vi "Autonomous Independent.vi"() -> ()   [LabVIEW 2014]
doc: "This VI is called when autonomous begins, and will automatically be terminated when autonomous ends. You can carry out timed or sensor driven robot movement independently without needing to return to the caller."
uses:
  <vilib>/Rock Robotics/WPI/Joystick/WPI_JoystickGetSetRefNum.vi
  <vilib>/Rock Robotics/Network Tables/SD Write Numeric Array.vi
  <vilib>/Rock Robotics/WPI/RobotDrive/WPI_RobotDriveGetSetRefNum.vi
  <vilib>/Rock Robotics/WPI/RobotDrive/WPI_RobotDriveMecanumDrive_Cartesian.vi
panel:
  out "Current Movement, for debugging":T1 {"Z Joystick Value" scale=-1.0..1.0; "Y Joystick Value" scale=1.0..-1.0; "X Joystick Value" scale=-1.0..1.0}
  in  "Array of robot movements":T2(array[cluster]) {"Z Joystick Value" scale=-1.0..1.0; "Y Joystick Value" scale=1.0..-1.0; "X Joystick Value" scale=-1.0..1.0}
  # "Be sure to right-click and choose Data Operations>>Make Current Value default if you want to save the array values with the VI"
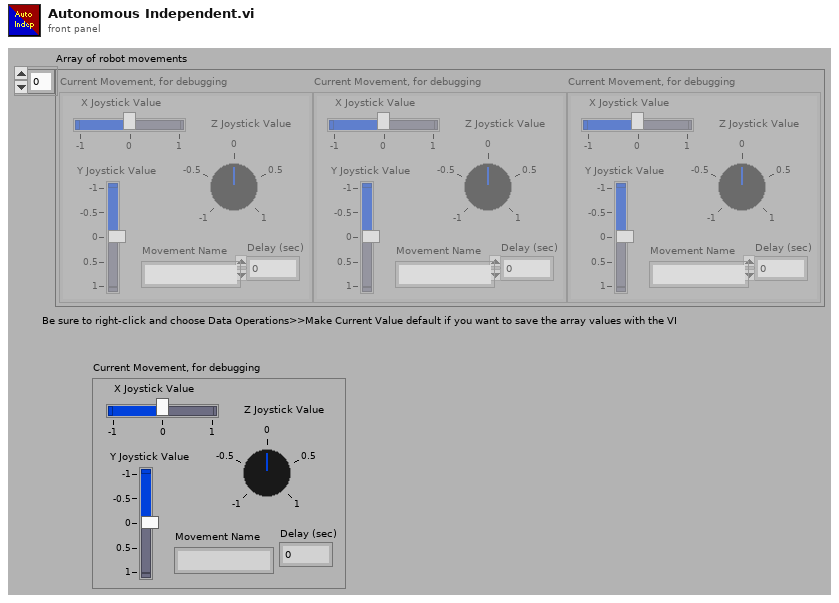
[diagram p1: front panel]
types:
  T1 = cluster{"X Joystick Value":dbl, "Y Joystick Value":dbl, "Z Joystick Value":dbl, "Delay (sec)":dbl, "Movement Name":string}
  T2 = cluster{"X Joystick Value":dbl, "Y Joystick Value":dbl, "Z Joystick Value":dbl, "Delay (sec)":dbl, "Movement Name":string}[]
  T3 = typedef "WPI_MotorControlDeviceRef.ctl" = cluster{"DeviceStatus":errorcluster, "Type":T4, "PWM":cluster{"Controller":T5, "PWM Channel":T6, "DeadBand":T7}, "CAN":cluster{"Device Number":u8, "Control Mode":T8, "Semaphore":T9, "Max Vout":dbl, "TalonSRX Control Mode":T10}, "Invert":bool, "TransformRef":T11, "InvTransformRef":T11}
  T4 = typedef "WPI_MotorControlType.ctl" = enum16{"PWM", "CAN", "CANTalonSRX"}
  T5 = typedef "FPGA_TypedefDigitalModule.ctl" = enum16{"Controller 1"}
  T6 = typedef "FPGA_DIOPWMChannel.ctl" = enum8{"PWM 0", "PWM 1", "PWM 2", "PWM 3", "PWM 4", "PWM 5", "PWM 6", "PWM 7", "PWM 8", "PWM 9", "PWM MXP 0", "PWM MXP 1", "PWM MXP 2", "PWM MXP 3", "PWM MXP 4", "PWM MXP 5", "PWM MXP 6", "PWM MXP 7", "PWM MXP 8", "PWM MXP 9", "Invalid"}
  T7 = typedef "WPI_PWMDeadband.ctl" = cluster{"Name":string, "maxPositivePwm":i32, "minPositivePwm":i32, "centerPwm":i32, "maxNegativePwm":i32, "minNegativePwm":i32, "angularRange":u16}
  T8 = typedef "WPI_CANJaguar_ControlMode.ctl" = enum8{"Percent VBus", "Current", "Speed", "Position", "Voltage"}
  T9 = typedef "Semaphore RefNum" = refnum<k1>
  T10 = typedef "WPI_CANTalonSRX_APIControlMode.ctl" = enum8{"Percent VBus", "Speed", "Position", "Slave", "Unchanged / Invalid"}
  T11 = typedef "WPI_PWMTransform_ConPane.ctl" = refnum<vi>
  T12 = typedef "WPI_RobotDriveDevRef.ctl" = cluster{"DevStatus":errorcluster, "Motors[]":T3[], "Square Inputs":bool, "Max Output":dbl}
  T13 = typedef "WPI_JoystickDevRef.ctl" = cluster{"Device":T14}
  T14 = typedef "WPI_JoystickDeviceEnum.ctl" = enum16{"USB 0", "USB 1", "USB 2", "USB 3", "USB 4", "USB 5"}
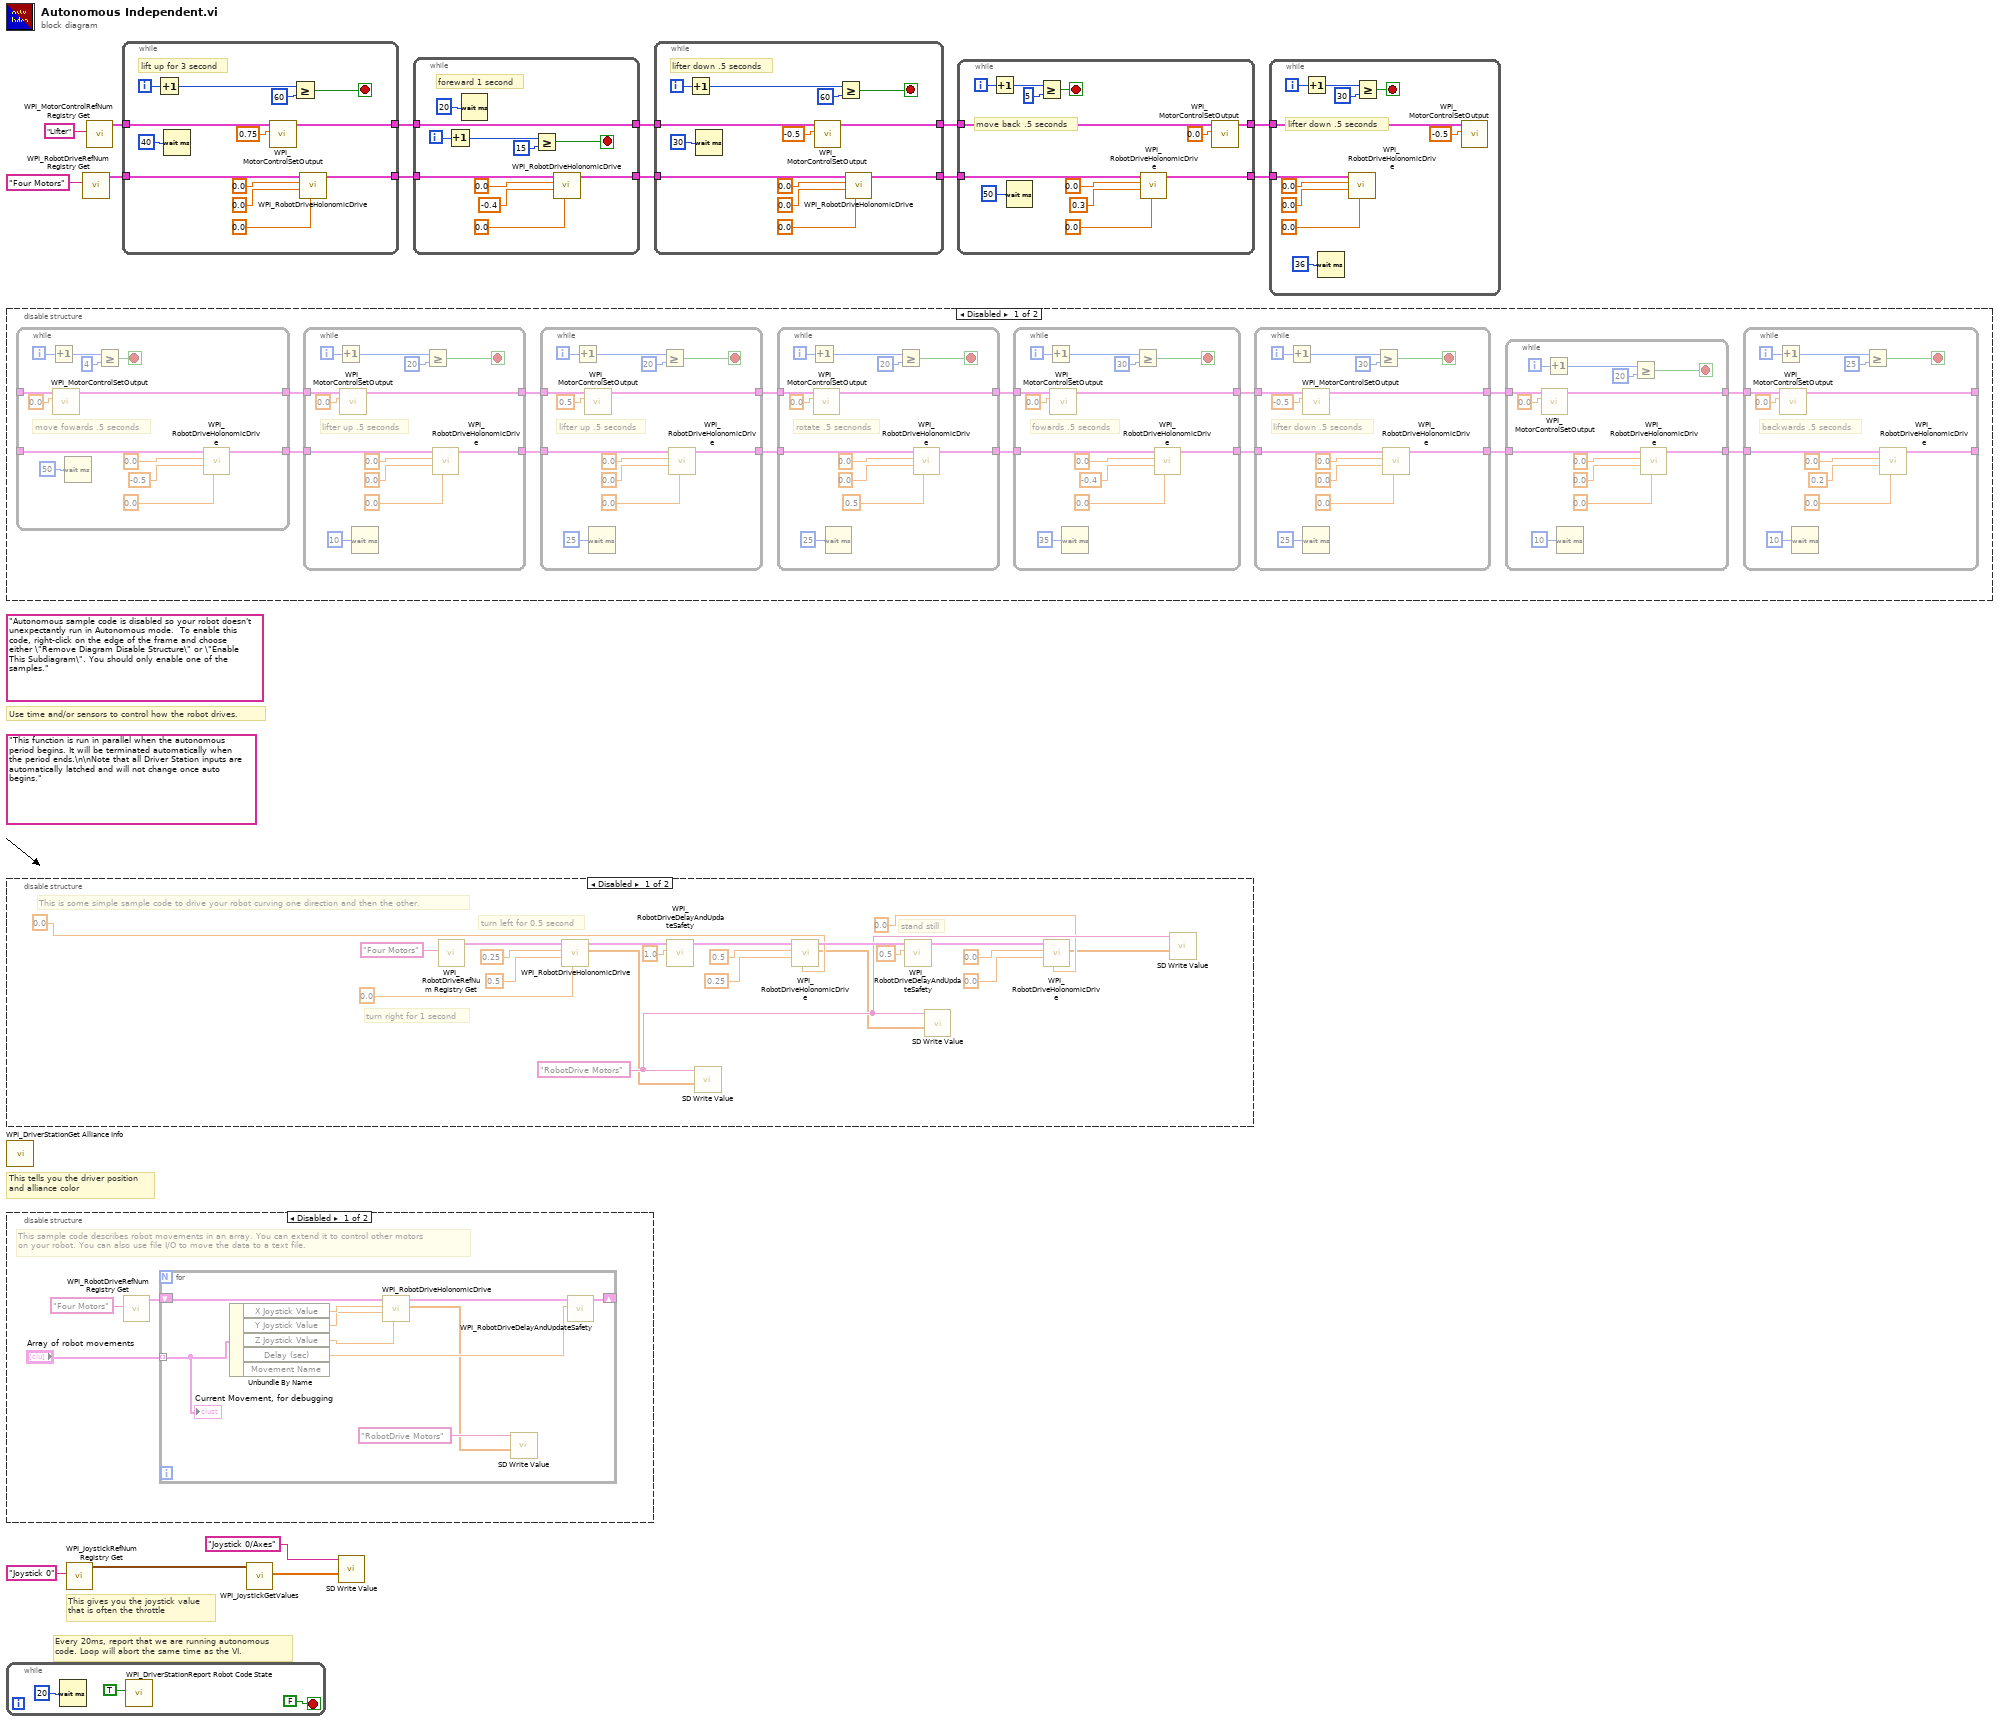
[diagram p0: block diagram]
diagram:
  (unwired) "Autonomous sample code is disabled so your robot doesn't unexpectantly run in Autonomous mode.  To enable this code, right-click on the edge of the frame and choose either \"Remove Diagram Disable Structure\" or \"Enable This Subdiagram\". You should only enable one of the samples."
  (unwired) "This function is run in parallel when the autonomous period begins. It will be terminated automatically when the period ends.\n\nNote that all Driver Station inputs are automatically latched and will not change once auto begins."
  # "Every 20ms, report that we are running autonomous\ncode. Loop will abort the same time as the VI."
  # "This gives you the joystick value\nthat is often the throttle"
  # "Use time and/or sensors to control how the robot drives."
  # "This tells you the driver position\nand alliance color"
  n1 = disable-structure shown="Disabled" {
    frame Disabled {
      n2 = while {
        tunnel: [w117] -> w19
        tunnel: [w113] -> w20
        tunnel: _ -> [w110]
        tunnel: _ -> [w109]
        i -> [w119]
        stop <- w118 stop-if-true
        # "move fowards .5 seconds"
        n3 = Increment(x=w119) -> (x+1=w120:i32)
        n4 = call <vilib>:"WPI_MotorControlSetOutput.vi"("Output"=0.0, "MotorControlDevRef"=w109) -> ("MotorControlDevRef"=w113:T3)  [unwired: 7 in, 2 out]
        n5 = Wait (ms)(milliseconds to wait=u32 50) -> ()  [unwired: 1 out]
        n6 = Greater Or Equal?(x=w120, y=4) -> (x >= y?=w118:bool)
        n7 = call-poly <vilib>:"WPI_RobotDriveHolonomicDrive.vi"("Rotation"=0.0, "Y"=-0.5 ("X"), "X"=0.0 ("Y"), "RobotDriveDevRef"=w110) -> ("RobotDriveDevRef"=w117:T12)  [unwired: 5 in, 2 out]
      }
      n8 = while {
        tunnel: [w130] -> w21
        tunnel: [w126] -> w22
        tunnel: w20 -> [w123]
        tunnel: w19 -> [w122]
        i -> [w132]
        stop <- w131 stop-if-true
        # "lifter up .5 seconds"
        n9 = Increment(x=w132) -> (x+1=w133:i32)
        n10 = call <vilib>:"WPI_MotorControlSetOutput.vi"("Output"=0.0, "MotorControlDevRef"=w123) -> ("MotorControlDevRef"=w126:T3)  [unwired: 7 in, 2 out]
        n11 = Wait (ms)(milliseconds to wait=u32 10) -> ()  [unwired: 1 out]
        n12 = Greater Or Equal?(x=w133, y=20) -> (x >= y?=w131:bool)
        n13 = call-poly <vilib>:"WPI_RobotDriveHolonomicDrive.vi"("Rotation"=0.0, "Y"=0.0 ("X"), "X"=0.0 ("Y"), "RobotDriveDevRef"=w122) -> ("RobotDriveDevRef"=w130:T12)  [unwired: 5 in, 2 out]
      }
      n14 = while {
        tunnel: [w104] -> w26
        tunnel: [w100] -> w25
        tunnel: w22 -> [w97]
        tunnel: w21 -> [w96]
        i -> [w106]
        stop <- w105 stop-if-true
        # "lifter up .5 seconds"
        n15 = Increment(x=w106) -> (x+1=w107:i32)
        n16 = call <vilib>:"WPI_MotorControlSetOutput.vi"("Output"=0.5, "MotorControlDevRef"=w97) -> ("MotorControlDevRef"=w100:T3)  [unwired: 7 in, 2 out]
        n17 = Wait (ms)(milliseconds to wait=u32 25) -> ()  [unwired: 1 out]
        n18 = Greater Or Equal?(x=w107, y=20) -> (x >= y?=w105:bool)
        n19 = call-poly <vilib>:"WPI_RobotDriveHolonomicDrive.vi"("Rotation"=0.0, "Y"=0.0 ("X"), "X"=0.0 ("Y"), "RobotDriveDevRef"=w96) -> ("RobotDriveDevRef"=w104:T12)  [unwired: 5 in, 2 out]
      }
      n20 = while {
        tunnel: w26 -> [w91]
        tunnel: [w90] -> w30
        tunnel: w25 -> [w86]
        tunnel: [w85] -> w29
        i -> [w93]
        stop <- w92 stop-if-true
        # "rotate .5 secnonds"
        n21 = Increment(x=w93) -> (x+1=w94:i32)
        n22 = call <vilib>:"WPI_MotorControlSetOutput.vi"("Output"=0.0, "MotorControlDevRef"=w86) -> ("MotorControlDevRef"=w85:T3)  [unwired: 7 in, 2 out]
        n23 = Wait (ms)(milliseconds to wait=u32 25) -> ()  [unwired: 1 out]
        n24 = Greater Or Equal?(x=w94, y=20) -> (x >= y?=w92:bool)
        n25 = call-poly <vilib>:"WPI_RobotDriveHolonomicDrive.vi"("Rotation"=0.5, "Y"=0.0 ("X"), "X"=0.0 ("Y"), "RobotDriveDevRef"=w91) -> ("RobotDriveDevRef"=w90:T12)  [unwired: 5 in, 2 out]
      }
      n26 = while {
        tunnel: w30 -> [w78]
        tunnel: [w77] -> w27
        tunnel: w29 -> [w73]
        tunnel: [w72] -> w28
        i -> [w80]
        stop <- w79 stop-if-true
        # "fowards .5 seconds"
        n27 = Increment(x=w80) -> (x+1=w81:i32)
        n28 = call <vilib>:"WPI_MotorControlSetOutput.vi"("Output"=0.0, "MotorControlDevRef"=w73) -> ("MotorControlDevRef"=w72:T3)  [unwired: 7 in, 2 out]
        n29 = Wait (ms)(milliseconds to wait=u32 35) -> ()  [unwired: 1 out]
        n30 = Greater Or Equal?(x=w81, y=30) -> (x >= y?=w79:bool)
        n31 = call-poly <vilib>:"WPI_RobotDriveHolonomicDrive.vi"("Rotation"=0.0, "Y"=-0.4 ("X"), "X"=0.0 ("Y"), "RobotDriveDevRef"=w78) -> ("RobotDriveDevRef"=w77:T12)  [unwired: 5 in, 2 out]
      }
      n32 = while {
        tunnel: w27 -> [w65]
        tunnel: [w64] -> w24
        tunnel: w28 -> [w60]
        tunnel: [w59] -> w23
        i -> [w67]
        stop <- w66 stop-if-true
        # "lifter down .5 seconds"
        n33 = Increment(x=w67) -> (x+1=w68:i32)
        n34 = call <vilib>:"WPI_MotorControlSetOutput.vi"("Output"=-0.5, "MotorControlDevRef"=w60) -> ("MotorControlDevRef"=w59:T3)  [unwired: 7 in, 2 out]
        n35 = Wait (ms)(milliseconds to wait=u32 25) -> ()  [unwired: 1 out]
        n36 = Greater Or Equal?(x=w68, y=30) -> (x >= y?=w66:bool)
        n37 = call-poly <vilib>:"WPI_RobotDriveHolonomicDrive.vi"("Rotation"=0.0, "Y"=0.0 ("X"), "X"=0.0 ("Y"), "RobotDriveDevRef"=w65) -> ("RobotDriveDevRef"=w64:T12)  [unwired: 5 in, 2 out]
      }
      n38 = while {
        tunnel: [w39] -> w17
        tunnel: [w35] -> w18
        tunnel: w24 -> [w32]
        tunnel: w23 -> [w31]
        i -> [w41]
        stop <- w40 stop-if-true
        n39 = call <vilib>:"WPI_MotorControlSetOutput.vi"("Output"=0.0, "MotorControlDevRef"=w31) -> ("MotorControlDevRef"=w35:T3)  [unwired: 7 in, 2 out]
        n40 = Increment(x=w41) -> (x+1=w42:i32)
        n41 = Wait (ms)(milliseconds to wait=u32 10) -> ()  [unwired: 1 out]
        n42 = Greater Or Equal?(x=w42, y=20) -> (x >= y?=w40:bool)
        n43 = call-poly <vilib>:"WPI_RobotDriveHolonomicDrive.vi"("Rotation"=0.0, "Y"=0.0 ("X"), "X"=0.0 ("Y"), "RobotDriveDevRef"=w32) -> ("RobotDriveDevRef"=w39:T12)  [unwired: 5 in, 2 out]
      }
      n44 = while {
        tunnel: [w52] -> _
        tunnel: [w48] -> _
        tunnel: w18 -> [w45]
        tunnel: w17 -> [w44]
        i -> [w54]
        stop <- w53 stop-if-true
        # "backwards .5 seconds"
        n45 = Increment(x=w54) -> (x+1=w55:i32)
        n46 = call <vilib>:"WPI_MotorControlSetOutput.vi"("Output"=0.0, "MotorControlDevRef"=w45) -> ("MotorControlDevRef"=w48:T3)  [unwired: 7 in, 2 out]
        n47 = Wait (ms)(milliseconds to wait=u32 10) -> ()  [unwired: 1 out]
        n48 = Greater Or Equal?(x=w55, y=25) -> (x >= y?=w53:bool)
        n49 = call-poly <vilib>:"WPI_RobotDriveHolonomicDrive.vi"("Rotation"=0.0, "Y"=0.2 ("X"), "X"=0.0 ("Y"), "RobotDriveDevRef"=w44) -> ("RobotDriveDevRef"=w52:T12)  [unwired: 5 in, 2 out]
      }
    }
    frame Enabled {
    }
  }
  n50 = disable-structure shown="Disabled" {
    frame Disabled {
      w141 = "RobotDrive Motors" ("Name")
      # "This is some simple sample code to drive your robot curving one direction and then the other."
      # "stand still"
      # "turn left for 0.5 second"
      # "turn right for 1 second"
      n51 = call <vilib>:"WPI_RobotDriveRefNum Registry Get.vi"("refnum name"="Four Motors") -> ("RobotDriveDevRef"=w142:T12)  [unwired: 1 in, 9 out]
      n52 = call-poly <vilib>:"WPI_RobotDriveHolonomicDrive.vi"("Rotation"=0.0, "Y"=0.5 ("X axis value"), "X"=0.25 ("X axis value"), "RobotDriveDevRef"=w142) -> ("Motor Values"=w137:dbl[], "RobotDriveDevRef"=w149:T12)  [unwired: 5 in, 1 out]
      n53 = call <vilib>:"WPI_RobotDriveDelayAndUpdateSafety.vi"("Delay (s)"=1.0, "RobotDriveDevRef"=w149) -> ("RobotDriveDevRef 2"=w148:T12)  [unwired: 8 in, 1 out]
      n54 = call-poly <vilib>:"SD Write Value.vi"("Numeric Array"=w137, "Name"=w141) -> ()  [unwired: 8 in, 2 out]
      n55 = call-poly <vilib>:"WPI_RobotDriveHolonomicDrive.vi"("Rotation"=0.0, "Y"=0.25 ("X axis value"), "X"=0.5 ("X axis value"), "RobotDriveDevRef"=w148) -> ("Motor Values"=w136:dbl[], "RobotDriveDevRef"=w147:T12)  [unwired: 5 in, 1 out]
      n56 = call <vilib>:"WPI_RobotDriveDelayAndUpdateSafety.vi"("Delay (s)"=0.5, "RobotDriveDevRef"=w147) -> ("RobotDriveDevRef 2"=w146:T12)  [unwired: 8 in, 1 out]
      n57 = call-poly <vilib>:"SD Write Value.vi"("Numeric Array"=w136, "Name"=w141) -> ()  [unwired: 8 in, 2 out]
      n58 = call-poly <vilib>:"WPI_RobotDriveHolonomicDrive.vi"("Rotation"=0.0 ("X axis value"), "Y"=0.0 ("X axis value"), "X"=0.0 ("X axis value"), "RobotDriveDevRef"=w146) -> ("Motor Values"=w135:dbl[])  [unwired: 5 in, 2 out]
      n59 = call-poly <vilib>:"SD Write Value.vi"("Numeric Array"=w135, "Name"=w141) -> ()  [unwired: 8 in, 2 out]
    }
    frame Enabled {
    }
  }
  n60 = call <vilib>:"WPI_DriverStationGet Alliance Info.vi"() -> ()  [unwired: 12 out]
  n61 = disable-structure shown="Disabled" {
    frame Disabled {
      # "This sample code describes robot movements in an array. You can extend it to control other motors\non your robot. You can also use file I/O to move the data to a text file."
      n62 = call <vilib>:"WPI_RobotDriveRefNum Registry Get.vi"("refnum name"="Four Motors") -> ("RobotDriveDevRef"=w157:T12)  [unwired: 1 in, 9 out]
      n63 = for {
        shift-right: [w165] -> _
        shift-left: w157 -> [w166]
        tunnel: "Array of robot movements" -> [w161] mode=indexing
        n64 = Unbundle By Name(w161) -> ("X Joystick Value"=w164:dbl, "Y Joystick Value"=w163:dbl, "Z Joystick Value"=w160:dbl, "Delay (sec)"=w162:dbl)  [unwired: 1 out]
        n65 = call-poly <vilib>:"WPI_RobotDriveHolonomicDrive.vi"("Rotation"=w160, "Y"=w163, "X"=w164, "RobotDriveDevRef"=w166) -> ("Motor Values"=w159:dbl[], "RobotDriveDevRef"=w167:T12)  [unwired: 5 in, 1 out]
        n66 = call-poly <vilib>:"SD Write Value.vi"("Numeric Array"=w159, "Name"="RobotDrive Motors") -> ()  [unwired: 8 in, 2 out]
        n67 = call <vilib>:"WPI_RobotDriveDelayAndUpdateSafety.vi"("Delay (s)"=w162, "RobotDriveDevRef"=w167) -> ("RobotDriveDevRef 2"=w165:T12)  [unwired: 8 in, 1 out]
        "Current Movement, for debugging" <- w161
      }
    }
    frame Enabled {
    }
  }
  n68 = while {
    stop <- FALSE stop-if-true
    n69 = Wait (ms)(milliseconds to wait=u32 20) -> ()  [unwired: 1 out]
    n70 = call <vilib>:"WPI_DriverStationReport Robot Code State.vi"("Autonomous"=TRUE) -> ()  [unwired: 10 in, 1 out]
  }
  n71 = call <vilib>:"WPI_JoystickRefNum Registry Get.vi"("refnum name"="Joystick 0") -> ("JoystickDevRef"=w15:T13)  [unwired: 1 in, 9 out]
  n72 = call <vilib>:"WPI_RobotDriveRefNum Registry Get.vi"("refnum name"="Four Motors") -> ("RobotDriveDevRef"=w8:T12)  [unwired: 1 in, 9 out]
  n73 = call <vilib>:"WPI_MotorControlRefNum Registry Get.vi"("refnum name"="Lifter") -> ("MotorControlDevRef"=w7:T3)  [unwired: 9 in, 1 out]
  n74 = while {
    tunnel: [w176] -> w10
    tunnel: [w174] -> w9
    tunnel: w8 -> [w173]
    tunnel: w7 -> [w172]
    i -> [w184]
    stop <- w181 stop-if-true
    # "lift up for 3 second"
    n75 = Increment(x=w184) -> (x+1=w183:i32)
    n76 = Wait (ms)(milliseconds to wait=u32 40) -> ()  [unwired: 1 out]
    n77 = call <vilib>:"WPI_MotorControlSetOutput.vi"("Output"=0.75, "MotorControlDevRef"=w172) -> ("MotorControlDevRef"=w174:T3)  [unwired: 7 in, 2 out]
    n78 = Greater Or Equal?(x=w183, y=60) -> (x >= y?=w181:bool)
    n79 = call-poly <vilib>:"WPI_RobotDriveHolonomicDrive.vi"("Rotation"=0.0, "Y"=0.0 ("X axis value"), "X"=0.0 ("X axis value"), "RobotDriveDevRef"=w173) -> ("RobotDriveDevRef"=w176:T12)  [unwired: 5 in, 2 out]
  }
  n80 = call <vilib>:"WPI_JoystickGetValues.vi"("JoystickDevRef"=w15) -> ("Axes"=w13:dbl[])  [unwired: 6 in, 4 out]
  n81 = call-poly <vilib>:"SD Write Value.vi"("Numeric Array"=w13, "Name"="Joystick 0/Axes") -> ()  [unwired: 8 in, 2 out]
  n82 = while {
    tunnel: [w187] -> w5
    tunnel: [w186] -> w6
    tunnel: w9 -> [w186]
    tunnel: w10 -> [w185]
    i -> [w195]
    stop <- w192 stop-if-true
    # "foreward 1 second"
    n83 = Increment(x=w195) -> (x+1=w194:i32)
    n84 = Wait (ms)(milliseconds to wait=u32 20) -> ()  [unwired: 1 out]
    n85 = Greater Or Equal?(x=w194, y=15) -> (x >= y?=w192:bool)
    n86 = call-poly <vilib>:"WPI_RobotDriveHolonomicDrive.vi"("Rotation"=0.0, "Y"=-0.4 ("X axis value"), "X"=0.0 ("X axis value"), "RobotDriveDevRef"=w185) -> ("RobotDriveDevRef"=w187:T12)  [unwired: 5 in, 2 out]
  }
  n87 = while {
    tunnel: [w200] -> w3
    tunnel: [w199] -> w4
    tunnel: w6 -> [w197]
    tunnel: w5 -> [w196]
    i -> [w208]
    stop <- w205 stop-if-true
    # "lifter down .5 seconds"
    n88 = Increment(x=w208) -> (x+1=w207:i32)
    n89 = Wait (ms)(milliseconds to wait=u32 30) -> ()  [unwired: 1 out]
    n90 = call <vilib>:"WPI_MotorControlSetOutput.vi"("Output"=-0.5, "MotorControlDevRef"=w197) -> ("MotorControlDevRef"=w199:T3)  [unwired: 7 in, 2 out]
    n91 = Greater Or Equal?(x=w207, y=60) -> (x >= y?=w205:bool)
    n92 = call-poly <vilib>:"WPI_RobotDriveHolonomicDrive.vi"("Rotation"=0.0, "Y"=0.0 ("X axis value"), "X"=0.0 ("X axis value"), "RobotDriveDevRef"=w196) -> ("RobotDriveDevRef"=w200:T12)  [unwired: 5 in, 2 out]
  }
  n93 = while {
    tunnel: w3 -> [w214]
    tunnel: w4 -> [w210]
    tunnel: [w211] -> w2
    tunnel: [w212] -> w1
    i -> [w221]
    stop <- w218 stop-if-true
    # "move back .5 seconds"
    n94 = Increment(x=w221) -> (x+1=w220:i32)
    n95 = Wait (ms)(milliseconds to wait=u32 50) -> ()  [unwired: 1 out]
    n96 = Greater Or Equal?(x=w220, y=5) -> (x >= y?=w218:bool)
    n97 = call-poly <vilib>:"WPI_RobotDriveHolonomicDrive.vi"("Rotation"=0.0, "Y"=0.3 ("X axis value"), "X"=0.0 ("X axis value"), "RobotDriveDevRef"=w214) -> ("RobotDriveDevRef"=w212:T12)  [unwired: 5 in, 2 out]
    n98 = call <vilib>:"WPI_MotorControlSetOutput.vi"("Output"=0.0, "MotorControlDevRef"=w210) -> ("MotorControlDevRef"=w211:T3)  [unwired: 7 in, 2 out]
  }
  n99 = while {
    tunnel: w2 -> [w225]
    tunnel: w1 -> [w224]
    i -> [w222]
    stop <- w223 stop-if-true
    # "lifter down .5 seconds"
    n100 = Increment(x=w222) -> (x+1=w227:i32)
    n101 = Wait (ms)(milliseconds to wait=u32 36) -> ()  [unwired: 1 out]
    n102 = call-poly <vilib>:"WPI_RobotDriveHolonomicDrive.vi"("Rotation"=0.0, "Y"=0.0 ("X"), "X"=0.0 ("Y"), "RobotDriveDevRef"=w224) -> ()  [unwired: 5 in, 3 out]
    n103 = Greater Or Equal?(x=w227, y=30) -> (x >= y?=w223:bool)
    n104 = call <vilib>:"WPI_MotorControlSetOutput.vi"("Output"=-0.5, "MotorControlDevRef"=w225) -> ()  [unwired: 7 in, 3 out]
  }
